vi "Lab Panel V4.88.vi"() -> ()   [LabVIEW 2013] (continued)
                    n1116 = Greater Or Equal?(x=w2161, y=w2154) -> (x >= y?=w2163:bool)
                    n1117 = case shown="True" w2163 {
                      tunnel: w2158 -> [w2173 _]
                      tunnel: w2157 -> [w2172 _]
                      tunnel: w2156 -> [w2171 _]
                      tunnel: w2155 -> [w2170 _]
                      frame True {
                        n1118 = stacked-sequence {
                          tunnel: w2173 -> [w2177 _]
                          tunnel: w2172 -> [w2175 w2181]
                          tunnel: w2171 -> [_ w2184]
                          tunnel: w2170 -> [w2174 _]
                          frame #0 {
                            n1119 = Build Array(w2175) -> (w2178:string[])
                            n1120 = Build Array(w2177) -> (w2176:dbl[])
                            n1121 = TDMS Write(0:w2174, 5:"TEST PASS", 7:w2178, 9:w2176) -> (15:w2180:errorcluster)  [unwired: 2 in, 3 out]
                            n1122 = local write "data file error"(w2180) -> ()
                          }
                          frame #1 {
                            n1123 = Bundle(cluster=w2184, "STATUS"=w2181) -> (w2182:T4)  [unwired: 2 in]
                            n1124 = local write "RESULT LAB02-1"(TRUE) -> ()
                            n1125 = local write "DISP LAB02-1"(w2182) -> ()
                          }
                        }
                      }
                      frame False {
                      }
                    }
                  }
                }
              }
              frame #3 {
                # "LAB02-2"
                n1126 = Less?(x=w2185, y=2) -> (x < y?=w2188:bool)
                n1127 = local read "DISP LAB02-2"() -> (w2190:T4)
                n1128 = Unbundle(w2190) -> ("STATUS"=w2191:string)  [unwired: 2 out]
                n1129 = Equal?(x=w2191, y="RUN") -> (x = y?=w2187:bool)
                n1130 = And(x=w2187, y=w2188) -> (x .and. y?=w2186:bool)
                n1131 = case shown="True" w2186 {
                  tunnel: w2190 -> [_ w2196]
                  tunnel: w2185 -> [_ w2200]
                  frame False {
                  }
                  frame True {
                    n1132 = local read "SET LAB02-2"() -> (w2202:T5)
                    n1133 = local read "TDMS LAB02-2"() -> (w2195:refnum<k34>)
                    n1134 = Unbundle(w2196) -> ("CYCLE"=w2201:dbl)  [unwired: 2 out]
                    n1135 = Unbundle(w2202) -> ("CYCLES"=w2193:dbl, "T-RISE mins"=w2199:dbl)  [unwired: 3 out]
                    n1136 = case shown="\"T-RISE TEST\"" w2200 {
                      tunnel: w2199 -> [_ _ w2209]
                      tunnel: [w2204 w2206 w2209] -> w2198
                      tunnel: w2193 -> [w2204 w2206 _]
                      tunnel: ["CHART PASS" "CYCLE PASS" "T-RISE PASS"] -> w2197
                      frame "CHART TEST", Default {
                      }
                      frame "CYCLE TEST" {
                      }
                      frame "T-RISE TEST" {
                      }
                    }
                    n1137 = Increment(x=w2193) -> (x+1=w2194:dbl)
                    n1138 = Greater Or Equal?(x=w2201, y=w2194) -> (x >= y?=w2203:bool)
                    n1139 = case shown="True" w2203 {
                      tunnel: w2198 -> [w2213 _]
                      tunnel: w2197 -> [w2212 _]
                      tunnel: w2196 -> [w2211 _]
                      tunnel: w2195 -> [w2210 _]
                      frame True {
                        n1140 = stacked-sequence {
                          tunnel: w2213 -> [w2217 _]
                          tunnel: w2212 -> [w2215 w2221]
                          tunnel: w2211 -> [_ w2224]
                          tunnel: w2210 -> [w2214 _]
                          frame #0 {
                            n1141 = Build Array(w2215) -> (w2218:string[])
                            n1142 = Build Array(w2217) -> (w2216:dbl[])
                            n1143 = TDMS Write(0:w2214, 5:"TEST PASS", 7:w2218, 9:w2216) -> (15:w2220:errorcluster)  [unwired: 2 in, 3 out]
                            n1144 = local write "data file error"(w2220) -> ()
                          }
                          frame #1 {
                            n1145 = Bundle(cluster=w2224, "STATUS"=w2221) -> (w2222:T4)  [unwired: 2 in]
                            n1146 = local write "RESULT LAB02-2"(TRUE) -> ()
                            n1147 = local write "DISP LAB02-2"(w2222) -> ()
                          }
                        }
                      }
                      frame False {
                      }
                    }
                  }
                }
              }
              frame #4 {
                # "LAB03-1"
                n1148 = Less?(x=w2225, y=2) -> (x < y?=w2228:bool)
                n1149 = local read "DISP LAB03-1"() -> (w2230:T4)
                n1150 = Unbundle(w2230) -> ("STATUS"=w2231:string)  [unwired: 2 out]
                n1151 = Equal?(x=w2231, y="RUN") -> (x = y?=w2227:bool)
                n1152 = And(x=w2227, y=w2228) -> (x .and. y?=w2226:bool)
                n1153 = case shown="True" w2226 {
                  tunnel: w2230 -> [_ w2236]
                  tunnel: w2225 -> [_ w2240]
                  frame False {
                  }
                  frame True {
                    n1154 = local read "SET LAB03-1"() -> (w2242:T5)
                    n1155 = local read "TDMS LAB03-1"() -> (w2235:refnum<k34>)
                    n1156 = Unbundle(w2236) -> ("CYCLE"=w2241:dbl)  [unwired: 2 out]
                    n1157 = Unbundle(w2242) -> ("CYCLES"=w2233:dbl, "T-RISE mins"=w2239:dbl)  [unwired: 3 out]
                    n1158 = case shown="\"T-RISE TEST\"" w2240 {
                      tunnel: w2239 -> [_ _ w2249]
                      tunnel: [w2244 w2246 w2249] -> w2238
                      tunnel: w2233 -> [w2244 w2246 _]
                      tunnel: ["CHART PASS" "CYCLE PASS" "T-RISE PASS"] -> w2237
                      frame "CHART TEST", Default {
                      }
                      frame "CYCLE TEST" {
                      }
                      frame "T-RISE TEST" {
                      }
                    }
                    n1159 = Increment(x=w2233) -> (x+1=w2234:dbl)
                    n1160 = Greater Or Equal?(x=w2241, y=w2234) -> (x >= y?=w2243:bool)
                    n1161 = case shown="True" w2243 {
                      tunnel: w2238 -> [w2253 _]
                      tunnel: w2237 -> [w2252 _]
                      tunnel: w2236 -> [w2251 _]
                      tunnel: w2235 -> [w2250 _]
                      frame True {
                        n1162 = stacked-sequence {
                          tunnel: w2253 -> [w2257 _]
                          tunnel: w2252 -> [w2255 w2261]
                          tunnel: w2251 -> [_ w2264]
                          tunnel: w2250 -> [w2254 _]
                          frame #0 {
                            n1163 = Build Array(w2255) -> (w2258:string[])
                            n1164 = Build Array(w2257) -> (w2256:dbl[])
                            n1165 = TDMS Write(0:w2254, 5:"TEST PASS", 7:w2258, 9:w2256) -> (15:w2260:errorcluster)  [unwired: 2 in, 3 out]
                            n1166 = local write "data file error"(w2260) -> ()
                          }
                          frame #1 {
                            n1167 = Bundle(cluster=w2264, "STATUS"=w2261) -> (w2262:T4)  [unwired: 2 in]
                            n1168 = local write "RESULT LAB03-1"(TRUE) -> ()
                            n1169 = local write "DISP LAB03-1"(w2262) -> ()
                          }
                        }
                      }
                      frame False {
                      }
                    }
                  }
                }
              }
              frame #5 {
                # "LAB03-2"
                n1170 = Less?(x=w2265, y=2) -> (x < y?=w2268:bool)
                n1171 = local read "DISP LAB03-2"() -> (w2270:T4)
                n1172 = Unbundle(w2270) -> ("STATUS"=w2271:string)  [unwired: 2 out]
                n1173 = Equal?(x=w2271, y="RUN") -> (x = y?=w2267:bool)
                n1174 = And(x=w2267, y=w2268) -> (x .and. y?=w2266:bool)
                n1175 = case shown="True" w2266 {
                  tunnel: w2270 -> [_ w2276]
                  tunnel: w2265 -> [_ w2280]
                  frame False {
                  }
                  frame True {
                    n1176 = local read "SET LAB03-2"() -> (w2282:T5)
                    n1177 = local read "TDMS LAB03-2"() -> (w2275:refnum<k34>)
                    n1178 = Unbundle(w2276) -> ("CYCLE"=w2281:dbl)  [unwired: 2 out]
                    n1179 = Unbundle(w2282) -> ("CYCLES"=w2273:dbl, "T-RISE mins"=w2279:dbl)  [unwired: 3 out]
                    n1180 = case shown="\"T-RISE TEST\"" w2280 {
                      tunnel: w2279 -> [_ _ w2289]
                      tunnel: [w2284 w2286 w2289] -> w2278
                      tunnel: w2273 -> [w2284 w2286 _]
                      tunnel: ["CHART PASS" "CYCLE PASS" "T-RISE PASS"] -> w2277
                      frame "CHART TEST", Default {
                      }
                      frame "CYCLE TEST" {
                      }
                      frame "T-RISE TEST" {
                      }
                    }
                    n1181 = Increment(x=w2273) -> (x+1=w2274:dbl)
                    n1182 = Greater Or Equal?(x=w2281, y=w2274) -> (x >= y?=w2283:bool)
                    n1183 = case shown="True" w2283 {
                      tunnel: w2278 -> [w2293 _]
                      tunnel: w2277 -> [w2292 _]
                      tunnel: w2276 -> [w2291 _]
                      tunnel: w2275 -> [w2290 _]
                      frame True {
                        n1184 = stacked-sequence {
                          tunnel: w2293 -> [w2297 _]
                          tunnel: w2292 -> [w2295 w2301]
                          tunnel: w2291 -> [_ w2304]
                          tunnel: w2290 -> [w2294 _]
                          frame #0 {
                            n1185 = Build Array(w2295) -> (w2298:string[])
                            n1186 = Build Array(w2297) -> (w2296:dbl[])
                            n1187 = TDMS Write(0:w2294, 5:"TEST PASS", 7:w2298, 9:w2296) -> (15:w2300:errorcluster)  [unwired: 2 in, 3 out]
                            n1188 = local write "data file error"(w2300) -> ()
                          }
                          frame #1 {
                            n1189 = Bundle(cluster=w2304, "STATUS"=w2301) -> (w2302:T4)  [unwired: 2 in]
                            n1190 = local write "RESULT LAB03-2"(TRUE) -> ()
                            n1191 = local write "DISP LAB03-2"(w2302) -> ()
                          }
                        }
                      }
                      frame False {
                      }
                    }
                  }
                }
              }
              frame #6 {
                # "LAB04-1"
                n1192 = Less?(x=w2305, y=2) -> (x < y?=w2308:bool)
                n1193 = local read "DISP LAB04-1"() -> (w2310:T4)
                n1194 = Unbundle(w2310) -> ("STATUS"=w2311:string)  [unwired: 2 out]
                n1195 = Equal?(x=w2311, y="RUN") -> (x = y?=w2307:bool)
                n1196 = And(x=w2307, y=w2308) -> (x .and. y?=w2306:bool)
                n1197 = case shown="True" w2306 {
                  tunnel: w2310 -> [_ w2316]
                  tunnel: w2305 -> [_ w2320]
                  frame False {
                  }
                  frame True {
                    n1198 = local read "SET LAB04-1"() -> (w2322:T5)
                    n1199 = local read "TDMS LAB04-1"() -> (w2315:refnum<k34>)
                    n1200 = Unbundle(w2316) -> ("CYCLE"=w2321:dbl)  [unwired: 2 out]
                    n1201 = Unbundle(w2322) -> ("CYCLES"=w2313:dbl, "T-RISE mins"=w2319:dbl)  [unwired: 3 out]
                    n1202 = case shown="\"T-RISE TEST\"" w2320 {
                      tunnel: w2319 -> [_ _ w2329]
                      tunnel: [w2324 w2326 w2329] -> w2318
                      tunnel: w2313 -> [w2324 w2326 _]
                      tunnel: ["CHART PASS" "CYCLE PASS" "T-RISE PASS"] -> w2317
                      frame "CHART TEST", Default {
                      }
                      frame "CYCLE TEST" {
                      }
                      frame "T-RISE TEST" {
                      }
                    }
                    n1203 = Increment(x=w2313) -> (x+1=w2314:dbl)
                    n1204 = Greater Or Equal?(x=w2321, y=w2314) -> (x >= y?=w2323:bool)
                    n1205 = case shown="True" w2323 {
                      tunnel: w2318 -> [w2333 _]
                      tunnel: w2317 -> [w2332 _]
                      tunnel: w2316 -> [w2331 _]
                      tunnel: w2315 -> [w2330 _]
                      frame True {
                        n1206 = stacked-sequence {
                          tunnel: w2333 -> [w2337 _]
                          tunnel: w2332 -> [w2335 w2341]
                          tunnel: w2331 -> [_ w2344]
                          tunnel: w2330 -> [w2334 _]
                          frame #0 {
                            n1207 = Build Array(w2335) -> (w2338:string[])
                            n1208 = Build Array(w2337) -> (w2336:dbl[])
                            n1209 = TDMS Write(0:w2334, 5:"TEST PASS", 7:w2338, 9:w2336) -> (15:w2340:errorcluster)  [unwired: 2 in, 3 out]
                            n1210 = local write "data file error"(w2340) -> ()
                          }
                          frame #1 {
                            n1211 = Bundle(cluster=w2344, "STATUS"=w2341) -> (w2342:T4)  [unwired: 2 in]
                            n1212 = local write "RESULT LAB04-1"(TRUE) -> ()
                            n1213 = local write "DISP LAB04-1"(w2342) -> ()
                          }
                        }
                      }
                      frame False {
                      }
                    }
                  }
                }
              }
              frame #7 {
                # "LAB04-2"
                n1214 = Less?(x=w2345, y=2) -> (x < y?=w2348:bool)
                n1215 = local read "DISP LAB04-2"() -> (w2350:T4)
                n1216 = Unbundle(w2350) -> ("STATUS"=w2351:string)  [unwired: 2 out]
                n1217 = Equal?(x=w2351, y="RUN") -> (x = y?=w2347:bool)
                n1218 = And(x=w2347, y=w2348) -> (x .and. y?=w2346:bool)
                n1219 = case shown="True" w2346 {
                  tunnel: w2350 -> [_ w2356]
                  tunnel: w2345 -> [_ w2360]
                  frame False {
                  }
                  frame True {
                    n1220 = local read "SET LAB04-2"() -> (w2362:T5)
                    n1221 = local read "TDMS LAB04-2"() -> (w2355:refnum<k34>)
                    n1222 = Unbundle(w2356) -> ("CYCLE"=w2361:dbl)  [unwired: 2 out]
                    n1223 = Unbundle(w2362) -> ("CYCLES"=w2353:dbl, "T-RISE mins"=w2359:dbl)  [unwired: 3 out]
                    n1224 = case shown="\"T-RISE TEST\"" w2360 {
                      tunnel: w2359 -> [_ _ w2369]
                      tunnel: [w2364 w2366 w2369] -> w2358
                      tunnel: w2353 -> [w2364 w2366 _]
                      tunnel: ["CHART PASS" "CYCLE PASS" "T-RISE PASS"] -> w2357
                      frame "CHART TEST", Default {
                      }
                      frame "CYCLE TEST" {
                      }
                      frame "T-RISE TEST" {
                      }
                    }
                    n1225 = Increment(x=w2353) -> (x+1=w2354:dbl)
                    n1226 = Greater Or Equal?(x=w2361, y=w2354) -> (x >= y?=w2363:bool)
                    n1227 = case shown="True" w2363 {
                      tunnel: w2358 -> [w2373 _]
                      tunnel: w2357 -> [w2372 _]
                      tunnel: w2356 -> [w2371 _]
                      tunnel: w2355 -> [w2370 _]
                      frame True {
                        n1228 = stacked-sequence {
                          tunnel: w2373 -> [w2377 _]
                          tunnel: w2372 -> [w2375 w2381]
                          tunnel: w2371 -> [_ w2384]
                          tunnel: w2370 -> [w2374 _]
                          frame #0 {
                            n1229 = Build Array(w2375) -> (w2378:string[])
                            n1230 = Build Array(w2377) -> (w2376:dbl[])
                            n1231 = TDMS Write(0:w2374, 5:"TEST PASS", 7:w2378, 9:w2376) -> (15:w2380:errorcluster)  [unwired: 2 in, 3 out]
                            n1232 = local write "data file error"(w2380) -> ()
                          }
                          frame #1 {
                            n1233 = Bundle(cluster=w2384, "STATUS"=w2381) -> (w2382:T4)  [unwired: 2 in]
                            n1234 = local write "RESULT LAB04-2"(TRUE) -> ()
                            n1235 = local write "DISP LAB04-2"(w2382) -> ()
                          }
                        }
                      }
                      frame False {
                      }
                    }
                  }
                }
              }
              frame #8 {
                # "LAB05-1"
                n1236 = Less?(x=w2385, y=2) -> (x < y?=w2388:bool)
                n1237 = local read "DISP LAB05-1"() -> (w2390:T4)
                n1238 = Unbundle(w2390) -> ("STATUS"=w2391:string)  [unwired: 2 out]
                n1239 = Equal?(x=w2391, y="RUN") -> (x = y?=w2387:bool)
                n1240 = And(x=w2387, y=w2388) -> (x .and. y?=w2386:bool)
                n1241 = case shown="True" w2386 {
                  tunnel: w2390 -> [_ w2396]
                  tunnel: w2385 -> [_ w2400]
                  frame False {
                  }
                  frame True {
                    n1242 = local read "SET LAB05-1"() -> (w2402:T5)
                    n1243 = local read "TDMS LAB05-1"() -> (w2395:refnum<k34>)
                    n1244 = Unbundle(w2396) -> ("CYCLE"=w2401:dbl)  [unwired: 2 out]
                    n1245 = Unbundle(w2402) -> ("CYCLES"=w2393:dbl, "T-RISE mins"=w2399:dbl)  [unwired: 3 out]
                    n1246 = case shown="\"T-RISE TEST\"" w2400 {
                      tunnel: w2399 -> [_ _ w2409]
                      tunnel: [w2404 w2406 w2409] -> w2398
                      tunnel: w2393 -> [w2404 w2406 _]
                      tunnel: ["CHART PASS" "CYCLE PASS" "T-RISE PASS"] -> w2397
                      frame "CHART TEST", Default {
                      }
                      frame "CYCLE TEST" {
                      }
                      frame "T-RISE TEST" {
                      }
                    }
                    n1247 = Increment(x=w2393) -> (x+1=w2394:dbl)
                    n1248 = Greater Or Equal?(x=w2401, y=w2394) -> (x >= y?=w2403:bool)
                    n1249 = case shown="True" w2403 {
                      tunnel: w2398 -> [w2413 _]
                      tunnel: w2397 -> [w2412 _]
                      tunnel: w2396 -> [w2411 _]
                      tunnel: w2395 -> [w2410 _]
                      frame True {
                        n1250 = stacked-sequence {
                          tunnel: w2413 -> [w2417 _]
                          tunnel: w2412 -> [w2415 w2421]
                          tunnel: w2411 -> [_ w2424]
                          tunnel: w2410 -> [w2414 _]
                          frame #0 {
                            n1251 = Build Array(w2415) -> (w2418:string[])
                            n1252 = Build Array(w2417) -> (w2416:dbl[])
                            n1253 = TDMS Write(0:w2414, 5:"TEST PASS", 7:w2418, 9:w2416) -> (15:w2420:errorcluster)  [unwired: 2 in, 3 out]
                            n1254 = local write "data file error"(w2420) -> ()
                          }
                          frame #1 {
                            n1255 = Bundle(cluster=w2424, "STATUS"=w2421) -> (w2422:T4)  [unwired: 2 in]
                            n1256 = local write "RESULT LAB05-1"(TRUE) -> ()
                            n1257 = local write "DISP LAB05-1"(w2422) -> ()
                          }
                        }
                      }
                      frame False {
                      }
                    }
                  }
                }
              }
              frame #9 {
                # "LAB05-2"
                n1258 = Less?(x=w2425, y=2) -> (x < y?=w2428:bool)
                n1259 = local read "DISP LAB05-2"() -> (w2430:T4)
                n1260 = Unbundle(w2430) -> ("STATUS"=w2431:string)  [unwired: 2 out]
                n1261 = Equal?(x=w2431, y="RUN") -> (x = y?=w2427:bool)
                n1262 = And(x=w2427, y=w2428) -> (x .and. y?=w2426:bool)
                n1263 = case shown="True" w2426 {
                  tunnel: w2430 -> [_ w2436]
                  tunnel: w2425 -> [_ w2440]
                  frame False {
                  }
                  frame True {
                    n1264 = local read "SET LAB05-2"() -> (w2442:T5)
                    n1265 = local read "TDMS LAB05-2"() -> (w2435:refnum<k34>)
                    n1266 = Unbundle(w2436) -> ("CYCLE"=w2441:dbl)  [unwired: 2 out]
                    n1267 = Unbundle(w2442) -> ("CYCLES"=w2433:dbl, "T-RISE mins"=w2439:dbl)  [unwired: 3 out]
                    n1268 = case shown="\"T-RISE TEST\"" w2440 {
                      tunnel: w2439 -> [_ _ w2449]
                      tunnel: [w2444 w2446 w2449] -> w2438
                      tunnel: w2433 -> [w2444 w2446 _]
                      tunnel: ["CHART PASS" "CYCLE PASS" "T-RISE PASS"] -> w2437
                      frame "CHART TEST", Default {
                      }
                      frame "CYCLE TEST" {
                      }
                      frame "T-RISE TEST" {
                      }
                    }
                    n1269 = Increment(x=w2433) -> (x+1=w2434:dbl)
                    n1270 = Greater Or Equal?(x=w2441, y=w2434) -> (x >= y?=w2443:bool)
                    n1271 = case shown="True" w2443 {
                      tunnel: w2438 -> [w2453 _]
                      tunnel: w2437 -> [w2452 _]
                      tunnel: w2436 -> [w2451 _]
                      tunnel: w2435 -> [w2450 _]
                      frame True {
                        n1272 = stacked-sequence {
                          tunnel: w2453 -> [w2457 _]
                          tunnel: w2452 -> [w2455 w2461]
                          tunnel: w2451 -> [_ w2464]
                          tunnel: w2450 -> [w2454 _]
                          frame #0 {
                            n1273 = Build Array(w2455) -> (w2458:string[])
                            n1274 = Build Array(w2457) -> (w2456:dbl[])
                            n1275 = TDMS Write(0:w2454, 5:"TEST PASS", 7:w2458, 9:w2456) -> (15:w2460:errorcluster)  [unwired: 2 in, 3 out]
                            n1276 = local write "data file error"(w2460) -> ()
                          }
                          frame #1 {
                            n1277 = Bundle(cluster=w2464, "STATUS"=w2461) -> (w2462:T4)  [unwired: 2 in]
                            n1278 = local write "RESULT LAB05-2"(TRUE) -> ()
                            n1279 = local write "DISP LAB05-2"(w2462) -> ()
                          }
                        }
                      }
                      frame False {
                      }
                    }
                  }
                }
              }
            }
          }
          frame #5 {
            # "check if test cycles reached for temperature rise test"
            n1280 = stacked-sequence {
              tunnel: w2494 -> [_ _ _ _ _ _ _ _ _ _]
              tunnel: w2493 -> [_ _ _ _ _ _ _ _ _ _]
              tunnel: w2492 -> [_ _ _ _ _ _ _ _ _ _]
              tunnel: w2491 -> [_ _ _ _ _ _ _ _ _ _]
              tunnel: w2490 -> [_ _ _ _ _ _ _ _ _ _]
              tunnel: w2489 -> [_ _ _ _ _ _ _ _ _ _]
              tunnel: w2488 -> [_ _ _ _ _ _ _ _ _ _]
              tunnel: w2487 -> [_ _ _ _ _ _ _ _ _ _]
              tunnel: w2486 -> [_ _ _ _ _ _ _ _ _ _]
              tunnel: w2485 -> [_ _ _ _ _ _ _ _ _ _]
              tunnel: w2484 -> [w2500 _ _ _ _ _ _ _ _ _]
              tunnel: w2474 -> [w2495 _ _ _ _ _ _ _ _ _]
              tunnel: w2483 -> [_ w2526 _ _ _ _ _ _ _ _]
              tunnel: w2482 -> [_ _ w2556 _ _ _ _ _ _ _]
              tunnel: w2481 -> [_ _ _ w2586 _ _ _ _ _ _]
              tunnel: w2480 -> [_ _ _ _ w2616 _ _ _ _ _]
              tunnel: w2479 -> [_ _ _ _ _ w2646 _ _ _ _]
              tunnel: w2478 -> [_ _ _ _ _ _ w2676 _ _ _]
              tunnel: w2477 -> [_ _ _ _ _ _ _ w2706 _ _]
              tunnel: w2476 -> [_ _ _ _ _ _ _ _ w2736 _]
              tunnel: w2475 -> [_ _ _ _ _ _ _ _ _ w2766]
              tunnel: w2473 -> [_ w2525 _ _ _ _ _ _ _ _]
              tunnel: w2472 -> [_ _ w2555 _ _ _ _ _ _ _]
              tunnel: w2471 -> [_ _ _ w2585 _ _ _ _ _ _]
              tunnel: w2470 -> [_ _ _ _ w2615 _ _ _ _ _]
              tunnel: w2469 -> [_ _ _ _ _ w2645 _ _ _ _]
              tunnel: w2468 -> [_ _ _ _ _ _ w2675 _ _ _]
              tunnel: w2467 -> [_ _ _ _ _ _ _ w2705 _ _]
              tunnel: w2466 -> [_ _ _ _ _ _ _ _ w2735 _]
              tunnel: w2465 -> [_ _ _ _ _ _ _ _ _ w2765]
              frame #0 {
                # "LAB01-1"
                n1281 = Equal?(x=w2500, y=2) -> (x = y?=w2498:bool)
                n1282 = local read "DISP LAB01-1"() -> (w2501:T4)
                n1283 = Unbundle(w2501) -> ("STATUS"=w2502:string)  [unwired: 2 out]
                n1284 = Equal?(x=w2502, y="RUN") -> (x = y?=w2497:bool)
                n1285 = And(x=w2497, y=w2498) -> (x .and. y?=w2496:bool)
                n1286 = case shown="True" w2496 {
                  tunnel: w2501 -> [_ w2505]
                  tunnel: w2495 -> [_ w2508]
                  frame False {
                  }
                  frame True {
                    n1287 = local read "SET LAB01-1"() -> (w2507:T5)
                    n1288 = local read "TDMS LAB01-1"() -> (w2504:refnum<k34>)
                    n1289 = Unbundle(w2505) -> ("CYCLE"=w2509:dbl)  [unwired: 2 out]
                    n1290 = Unbundle(w2507) -> ("T-RISE mins"=w2506:dbl)  [unwired: 4 out]
                    n1291 = Greater Or Equal?(x=w2509, y=w2508) -> (x >= y?=w2510:bool)
                    n1292 = case shown="True" w2510 {
                      tunnel: w2506 -> [w2513 _]
                      tunnel: w2505 -> [w2512 _]
                      tunnel: w2504 -> [w2511 _]
                      frame True {
                        n1293 = stacked-sequence {
                          tunnel: w2513 -> [w2516 _]
                          tunnel: w2512 -> [_ w2521]
                          tunnel: w2511 -> [w2514 _]
                          frame #0 {
                            n1294 = Build Array("T-RISE") -> (w2518:string[])
                            n1295 = Build Array(w2516) -> (w2517:dbl[])
                            n1296 = TDMS Write(0:w2514, 5:"TEST PASS", 7:w2518, 9:w2517) -> (15:w2520:errorcluster)  [unwired: 2 in, 3 out]
                            n1297 = local write "data file error"(w2520) -> ()
                          }
                          frame #1 {
                            n1298 = Bundle(cluster=w2521, "STATUS"="T-RISE PASS") -> (w2523:T4)  [unwired: 2 in]
                            n1299 = local write "RESULT LAB01-1"(TRUE) -> ()
                            n1300 = local write "DISP LAB01-1"(w2523) -> ()
                          }
                        }
                      }
                      frame False {
                      }
                    }
                  }
                }
              }
              frame #1 {
                # "LAB01-2"
                n1301 = Equal?(x=w2526, y=2) -> (x = y?=w2529:bool)
                n1302 = local read "DISP LAB01-2"() -> (w2531:T4)
                n1303 = Unbundle(w2531) -> ("STATUS"=w2532:string)  [unwired: 2 out]
                n1304 = Equal?(x=w2532, y="RUN") -> (x = y?=w2528:bool)
                n1305 = And(x=w2528, y=w2529) -> (x .and. y?=w2527:bool)
                n1306 = case shown="True" w2527 {
                  tunnel: w2531 -> [_ w2535]
                  tunnel: w2525 -> [_ w2538]
                  frame False {
                  }
                  frame True {
                    n1307 = local read "SET LAB01-2"() -> (w2537:T5)
                    n1308 = local read "TDMS LAB01-2"() -> (w2534:refnum<k34>)
                    n1309 = Unbundle(w2535) -> ("CYCLE"=w2539:dbl)  [unwired: 2 out]
                    n1310 = Unbundle(w2537) -> ("T-RISE mins"=w2536:dbl)  [unwired: 4 out]
                    n1311 = Greater Or Equal?(x=w2539, y=w2538) -> (x >= y?=w2540:bool)
                    n1312 = case shown="True" w2540 {
                      tunnel: w2536 -> [w2543 _]
                      tunnel: w2535 -> [w2542 _]
                      tunnel: w2534 -> [w2541 _]
                      frame True {
                        n1313 = stacked-sequence {
                          tunnel: w2543 -> [w2546 _]
                          tunnel: w2542 -> [_ w2551]
                          tunnel: w2541 -> [w2544 _]
                          frame #0 {
                            n1314 = Build Array("T-RISE") -> (w2548:string[])
                            n1315 = Build Array(w2546) -> (w2547:dbl[])
                            n1316 = TDMS Write(0:w2544, 5:"TEST PASS", 7:w2548, 9:w2547) -> (15:w2550:errorcluster)  [unwired: 2 in, 3 out]
                            n1317 = local write "data file error"(w2550) -> ()
                          }
                          frame #1 {
                            n1318 = Bundle(cluster=w2551, "STATUS"="T-RISE PASS") -> (w2553:T4)  [unwired: 2 in]
                            n1319 = local write "RESULT LAB01-2"(TRUE) -> ()
                            n1320 = local write "DISP LAB01-2"(w2553) -> ()
                          }
                        }
                      }
                      frame False {
                      }
                    }
                  }
                }
              }
              frame #2 {
                # "LAB02-1"
                n1321 = Equal?(x=w2556, y=2) -> (x = y?=w2559:bool)
                n1322 = local read "DISP LAB02-1"() -> (w2561:T4)
                n1323 = Unbundle(w2561) -> ("STATUS"=w2562:string)  [unwired: 2 out]
                n1324 = Equal?(x=w2562, y="RUN") -> (x = y?=w2558:bool)
                n1325 = And(x=w2558, y=w2559) -> (x .and. y?=w2557:bool)
                n1326 = case shown="True" w2557 {
                  tunnel: w2561 -> [_ w2565]
                  tunnel: w2555 -> [_ w2568]
                  frame False {
                  }
                  frame True {
                    n1327 = local read "SET LAB02-1"() -> (w2567:T5)
                    n1328 = local read "TDMS LAB02-1"() -> (w2564:refnum<k34>)
                    n1329 = Unbundle(w2565) -> ("CYCLE"=w2569:dbl)  [unwired: 2 out]
                    n1330 = Unbundle(w2567) -> ("T-RISE mins"=w2566:dbl)  [unwired: 4 out]
                    n1331 = Greater Or Equal?(x=w2569, y=w2568) -> (x >= y?=w2570:bool)
                    n1332 = case shown="True" w2570 {
                      tunnel: w2566 -> [w2573 _]
                      tunnel: w2565 -> [w2572 _]
                      tunnel: w2564 -> [w2571 _]
                      frame True {
                        n1333 = stacked-sequence {
                          tunnel: w2573 -> [w2576 _]
                          tunnel: w2572 -> [_ w2581]
                          tunnel: w2571 -> [w2574 _]
                          frame #0 {
                            n1334 = Build Array("T-RISE") -> (w2578:string[])
                            n1335 = Build Array(w2576) -> (w2577:dbl[])
                            n1336 = TDMS Write(0:w2574, 5:"TEST PASS", 7:w2578, 9:w2577) -> (15:w2580:errorcluster)  [unwired: 2 in, 3 out]
                            n1337 = local write "data file error"(w2580) -> ()
                          }
                          frame #1 {
                            n1338 = Bundle(cluster=w2581, "STATUS"="T-RISE PASS") -> (w2583:T4)  [unwired: 2 in]
                            n1339 = local write "RESULT LAB02-1"(TRUE) -> ()
                            n1340 = local write "DISP LAB02-1"(w2583) -> ()
                          }
                        }
                      }
                      frame False {
                      }
                    }
                  }
                }
              }
              frame #3 {
                # "LAB02-2"
                n1341 = Equal?(x=w2586, y=2) -> (x = y?=w2589:bool)
                n1342 = local read "DISP LAB02-2"() -> (w2591:T4)
                n1343 = Unbundle(w2591) -> ("STATUS"=w2592:string)  [unwired: 2 out]
                n1344 = Equal?(x=w2592, y="RUN") -> (x = y?=w2588:bool)
                n1345 = And(x=w2588, y=w2589) -> (x .and. y?=w2587:bool)
                n1346 = case shown="True" w2587 {
                  tunnel: w2591 -> [_ w2595]
                  tunnel: w2585 -> [_ w2598]
                  frame False {
                  }
                  frame True {
                    n1347 = local read "SET LAB02-2"() -> (w2597:T5)
                    n1348 = local read "TDMS LAB02-2"() -> (w2594:refnum<k34>)
                    n1349 = Unbundle(w2595) -> ("CYCLE"=w2599:dbl)  [unwired: 2 out]
                    n1350 = Unbundle(w2597) -> ("T-RISE mins"=w2596:dbl)  [unwired: 4 out]
                    n1351 = Greater Or Equal?(x=w2599, y=w2598) -> (x >= y?=w2600:bool)
                    n1352 = case shown="True" w2600 {
                      tunnel: w2596 -> [w2603 _]
                      tunnel: w2595 -> [w2602 _]
                      tunnel: w2594 -> [w2601 _]
                      frame True {
                        n1353 = stacked-sequence {
                          tunnel: w2603 -> [w2606 _]
                          tunnel: w2602 -> [_ w2611]
                          tunnel: w2601 -> [w2604 _]
                          frame #0 {
                            n1354 = Build Array("T-RISE") -> (w2608:string[])
                            n1355 = Build Array(w2606) -> (w2607:dbl[])
                            n1356 = TDMS Write(0:w2604, 5:"TEST PASS", 7:w2608, 9:w2607) -> (15:w2610:errorcluster)  [unwired: 2 in, 3 out]
                            n1357 = local write "data file error"(w2610) -> ()
                          }
                          frame #1 {
                            n1358 = Bundle(cluster=w2611, "STATUS"="T-RISE PASS") -> (w2613:T4)  [unwired: 2 in]
                            n1359 = local write "RESULT LAB02-2"(TRUE) -> ()
                            n1360 = local write "DISP LAB02-2"(w2613) -> ()
                          }
                        }
                      }
                      frame False {
                      }
                    }
                  }
                }
              }
              frame #4 {
                # "LAB03-1"
                n1361 = Equal?(x=w2616, y=2) -> (x = y?=w2619:bool)
                n1362 = local read "DISP LAB03-1"() -> (w2621:T4)
                n1363 = Unbundle(w2621) -> ("STATUS"=w2622:string)  [unwired: 2 out]
                n1364 = Equal?(x=w2622, y="RUN") -> (x = y?=w2618:bool)
                n1365 = And(x=w2618, y=w2619) -> (x .and. y?=w2617:bool)
                n1366 = case shown="True" w2617 {
                  tunnel: w2621 -> [_ w2625]
                  tunnel: w2615 -> [_ w2628]
                  frame False {
                  }
                  frame True {
                    n1367 = local read "SET LAB03-1"() -> (w2627:T5)
                    n1368 = local read "TDMS LAB03-1"() -> (w2624:refnum<k34>)
                    n1369 = Unbundle(w2625) -> ("CYCLE"=w2629:dbl)  [unwired: 2 out]
                    n1370 = Unbundle(w2627) -> ("T-RISE mins"=w2626:dbl)  [unwired: 4 out]
                    n1371 = Greater Or Equal?(x=w2629, y=w2628) -> (x >= y?=w2630:bool)
                    n1372 = case shown="True" w2630 {
                      tunnel: w2626 -> [w2633 _]
                      tunnel: w2625 -> [w2632 _]
                      tunnel: w2624 -> [w2631 _]
                      frame True {
                        n1373 = stacked-sequence {
                          tunnel: w2633 -> [w2636 _]
                          tunnel: w2632 -> [_ w2641]
                          tunnel: w2631 -> [w2634 _]
                          frame #0 {
                            n1374 = Build Array("T-RISE") -> (w2638:string[])
                            n1375 = Build Array(w2636) -> (w2637:dbl[])
                            n1376 = TDMS Write(0:w2634, 5:"TEST PASS", 7:w2638, 9:w2637) -> (15:w2640:errorcluster)  [unwired: 2 in, 3 out]
                            n1377 = local write "data file error"(w2640) -> ()
                          }
                          frame #1 {
                            n1378 = Bundle(cluster=w2641, "STATUS"="T-RISE PASS") -> (w2643:T4)  [unwired: 2 in]
                            n1379 = local write "RESULT LAB03-1"(TRUE) -> ()
                            n1380 = local write "DISP LAB03-1"(w2643) -> ()
                          }
                        }
                      }
                      frame False {
                      }
                    }
                  }
                }
              }
              frame #5 {
                # "LAB03-2"
                n1381 = Equal?(x=w2646, y=2) -> (x = y?=w2649:bool)
                n1382 = local read "DISP LAB03-2"() -> (w2651:T4)
                n1383 = Unbundle(w2651) -> ("STATUS"=w2652:string)  [unwired: 2 out]
                n1384 = Equal?(x=w2652, y="RUN") -> (x = y?=w2648:bool)
                n1385 = And(x=w2648, y=w2649) -> (x .and. y?=w2647:bool)
                n1386 = case shown="True" w2647 {
                  tunnel: w2651 -> [_ w2655]
                  tunnel: w2645 -> [_ w2658]
                  frame False {
                  }
                  frame True {
                    n1387 = local read "SET LAB03-2"() -> (w2657:T5)
                    n1388 = local read "TDMS LAB03-2"() -> (w2654:refnum<k34>)
                    n1389 = Unbundle(w2655) -> ("CYCLE"=w2659:dbl)  [unwired: 2 out]
                    n1390 = Unbundle(w2657) -> ("T-RISE mins"=w2656:dbl)  [unwired: 4 out]
                    n1391 = Greater Or Equal?(x=w2659, y=w2658) -> (x >= y?=w2660:bool)
                    n1392 = case shown="True" w2660 {
                      tunnel: w2656 -> [w2663 _]
                      tunnel: w2655 -> [w2662 _]
                      tunnel: w2654 -> [w2661 _]
                      frame True {
                        n1393 = stacked-sequence {
                          tunnel: w2663 -> [w2666 _]
                          tunnel: w2662 -> [_ w2671]
                          tunnel: w2661 -> [w2664 _]
                          frame #0 {
                            n1394 = Build Array("T-RISE") -> (w2668:string[])
                            n1395 = Build Array(w2666) -> (w2667:dbl[])
                            n1396 = TDMS Write(0:w2664, 5:"TEST PASS", 7:w2668, 9:w2667) -> (15:w2670:errorcluster)  [unwired: 2 in, 3 out]
                            n1397 = local write "data file error"(w2670) -> ()
                          }
                          frame #1 {
                            n1398 = Bundle(cluster=w2671, "STATUS"="T-RISE PASS") -> (w2673:T4)  [unwired: 2 in]
                            n1399 = local write "RESULT LAB03-2"(TRUE) -> ()
                            n1400 = local write "DISP LAB03-2"(w2673) -> ()
                          }
                        }
                      }
                      frame False {
                      }
                    }
                  }
                }
              }
              frame #6 {
                # "LAB04-1"
                n1401 = Equal?(x=w2676, y=2) -> (x = y?=w2679:bool)
                n1402 = local read "DISP LAB04-1"() -> (w2681:T4)
                n1403 = Unbundle(w2681) -> ("STATUS"=w2682:string)  [unwired: 2 out]
                n1404 = Equal?(x=w2682, y="RUN") -> (x = y?=w2678:bool)
                n1405 = And(x=w2678, y=w2679) -> (x .and. y?=w2677:bool)
                n1406 = case shown="True" w2677 {
                  tunnel: w2681 -> [_ w2685]
                  tunnel: w2675 -> [_ w2688]
                  frame False {
                  }
                  frame True {
                    n1407 = local read "SET LAB04-1"() -> (w2687:T5)
                    n1408 = local read "TDMS LAB04-1"() -> (w2684:refnum<k34>)
                    n1409 = Unbundle(w2685) -> ("CYCLE"=w2689:dbl)  [unwired: 2 out]
                    n1410 = Unbundle(w2687) -> ("T-RISE mins"=w2686:dbl)  [unwired: 4 out]
                    n1411 = Greater Or Equal?(x=w2689, y=w2688) -> (x >= y?=w2690:bool)
                    n1412 = case shown="True" w2690 {
                      tunnel: w2686 -> [w2693 _]
                      tunnel: w2685 -> [w2692 _]
                      tunnel: w2684 -> [w2691 _]
                      frame True {
                        n1413 = stacked-sequence {
                          tunnel: w2693 -> [w2696 _]
                          tunnel: w2692 -> [_ w2701]
                          tunnel: w2691 -> [w2694 _]
                          frame #0 {
                            n1414 = Build Array("T-RISE") -> (w2698:string[])
                            n1415 = Build Array(w2696) -> (w2697:dbl[])
                            n1416 = TDMS Write(0:w2694, 5:"TEST PASS", 7:w2698, 9:w2697) -> (15:w2700:errorcluster)  [unwired: 2 in, 3 out]
                            n1417 = local write "data file error"(w2700) -> ()
                          }
                          frame #1 {
                            n1418 = Bundle(cluster=w2701, "STATUS"="T-RISE PASS") -> (w2703:T4)  [unwired: 2 in]
                            n1419 = local write "RESULT LAB04-1"(TRUE) -> ()
                            n1420 = local write "DISP LAB04-1"(w2703) -> ()
                          }
                        }
                      }
                      frame False {
                      }
                    }
                  }
                }
              }
              frame #7 {
                # "LAB04-2"
                n1421 = Equal?(x=w2706, y=2) -> (x = y?=w2709:bool)
                n1422 = local read "DISP LAB04-2"() -> (w2711:T4)
                n1423 = Unbundle(w2711) -> ("STATUS"=w2712:string)  [unwired: 2 out]
                n1424 = Equal?(x=w2712, y="RUN") -> (x = y?=w2708:bool)
                n1425 = And(x=w2708, y=w2709) -> (x .and. y?=w2707:bool)
                n1426 = case shown="True" w2707 {
                  tunnel: w2711 -> [_ w2715]
                  tunnel: w2705 -> [_ w2718]
                  frame False {
                  }
                  frame True {
                    n1427 = local read "SET LAB04-2"() -> (w2717:T5)
                    n1428 = local read "TDMS LAB04-2"() -> (w2714:refnum<k34>)
                    n1429 = Unbundle(w2715) -> ("CYCLE"=w2719:dbl)  [unwired: 2 out]
                    n1430 = Unbundle(w2717) -> ("T-RISE mins"=w2716:dbl)  [unwired: 4 out]
                    n1431 = Greater Or Equal?(x=w2719, y=w2718) -> (x >= y?=w2720:bool)
                    n1432 = case shown="True" w2720 {
                      tunnel: w2716 -> [w2723 _]
                      tunnel: w2715 -> [w2722 _]
                      tunnel: w2714 -> [w2721 _]
                      frame True {
                        n1433 = stacked-sequence {
                          tunnel: w2723 -> [w2726 _]
                          tunnel: w2722 -> [_ w2731]
                          tunnel: w2721 -> [w2724 _]
                          frame #0 {
                            n1434 = Build Array("T-RISE") -> (w2728:string[])
                            n1435 = Build Array(w2726) -> (w2727:dbl[])
                            n1436 = TDMS Write(0:w2724, 5:"TEST PASS", 7:w2728, 9:w2727) -> (15:w2730:errorcluster)  [unwired: 2 in, 3 out]
                            n1437 = local write "data file error"(w2730) -> ()
                          }
                          frame #1 {
                            n1438 = Bundle(cluster=w2731, "STATUS"="T-RISE PASS") -> (w2733:T4)  [unwired: 2 in]
                            n1439 = local write "RESULT LAB04-2"(TRUE) -> ()
                            n1440 = local write "DISP LAB04-2"(w2733) -> ()
                          }
                        }
                      }
                      frame False {
                      }
                    }
                  }
                }
              }
              frame #8 {
                # "LAB05-1"
                n1441 = Equal?(x=w2736, y=2) -> (x = y?=w2739:bool)
                n1442 = local read "DISP LAB05-1"() -> (w2741:T4)
                n1443 = Unbundle(w2741) -> ("STATUS"=w2742:string)  [unwired: 2 out]
                n1444 = Equal?(x=w2742, y="RUN") -> (x = y?=w2738:bool)
                n1445 = And(x=w2738, y=w2739) -> (x .and. y?=w2737:bool)
                n1446 = case shown="True" w2737 {
                  tunnel: w2741 -> [_ w2745]
                  tunnel: w2735 -> [_ w2748]
                  frame False {
                  }
                  frame True {
                    n1447 = local read "SET LAB05-1"() -> (w2747:T5)
                    n1448 = local read "TDMS LAB05-1"() -> (w2744:refnum<k34>)
                    n1449 = Unbundle(w2745) -> ("CYCLE"=w2749:dbl)  [unwired: 2 out]
                    n1450 = Unbundle(w2747) -> ("T-RISE mins"=w2746:dbl)  [unwired: 4 out]
                    n1451 = Greater Or Equal?(x=w2749, y=w2748) -> (x >= y?=w2750:bool)
                    n1452 = case shown="True" w2750 {
                      tunnel: w2746 -> [w2753 _]
                      tunnel: w2745 -> [w2752 _]
                      tunnel: w2744 -> [w2751 _]
                      frame True {
                        n1453 = stacked-sequence {
                          tunnel: w2753 -> [w2756 _]
                          tunnel: w2752 -> [_ w2761]
                          tunnel: w2751 -> [w2754 _]
                          frame #0 {
                            n1454 = Build Array("T-RISE") -> (w2758:string[])
                            n1455 = Build Array(w2756) -> (w2757:dbl[])
                            n1456 = TDMS Write(0:w2754, 5:"TEST PASS", 7:w2758, 9:w2757) -> (15:w2760:errorcluster)  [unwired: 2 in, 3 out]
                            n1457 = local write "data file error"(w2760) -> ()
                          }
                          frame #1 {
                            n1458 = Bundle(cluster=w2761, "STATUS"="T-RISE PASS") -> (w2763:T4)  [unwired: 2 in]
                            n1459 = local write "RESULT LAB05-1"(TRUE) -> ()
                            n1460 = local write "DISP LAB05-1"(w2763) -> ()
                          }
                        }
                      }
                      frame False {
                      }
                    }
                  }
                }
              }
              frame #9 {
                # "LAB05-2"
                n1461 = Equal?(x=w2766, y=2) -> (x = y?=w2769:bool)
                n1462 = local read "DISP LAB05-2"() -> (w2771:T4)
                n1463 = Unbundle(w2771) -> ("STATUS"=w2772:string)  [unwired: 2 out]
                n1464 = Equal?(x=w2772, y="RUN") -> (x = y?=w2768:bool)
                n1465 = And(x=w2768, y=w2769) -> (x .and. y?=w2767:bool)
                n1466 = case shown="True" w2767 {
                  tunnel: w2771 -> [_ w2775]
                  tunnel: w2765 -> [_ w2778]
                  frame False {
                  }
                  frame True {
                    n1467 = local read "SET LAB05-2"() -> (w2777:T5)
                    n1468 = local read "TDMS LAB05-2"() -> (w2774:refnum<k34>)
                    n1469 = Unbundle(w2775) -> ("CYCLE"=w2779:dbl)  [unwired: 2 out]
                    n1470 = Unbundle(w2777) -> ("T-RISE mins"=w2776:dbl)  [unwired: 4 out]
                    n1471 = Greater Or Equal?(x=w2779, y=w2778) -> (x >= y?=w2780:bool)
                    n1472 = case shown="True" w2780 {
                      tunnel: w2776 -> [w2783 _]
                      tunnel: w2775 -> [w2782 _]
                      tunnel: w2774 -> [w2781 _]
                      frame True {
                        n1473 = stacked-sequence {
                          tunnel: w2783 -> [w2786 _]
                          tunnel: w2782 -> [_ w2791]
                          tunnel: w2781 -> [w2784 _]
                          frame #0 {
                            n1474 = Build Array("T-RISE") -> (w2788:string[])
                            n1475 = Build Array(w2786) -> (w2787:dbl[])
                            n1476 = TDMS Write(0:w2784, 5:"TEST PASS", 7:w2788, 9:w2787) -> (15:w2790:errorcluster)  [unwired: 2 in, 3 out]
                            n1477 = local write "data file error"(w2790) -> ()
                          }
                          frame #1 {
                            n1478 = Bundle(cluster=w2791, "STATUS"="T-RISE PASS") -> (w2793:T4)  [unwired: 2 in]
